vi "dataFGV.vi"(7 "Enum":T1=enum."write data out", 8 "error in (no error)":errorcluster, 10 "DataOut":T3, 11 "DataIn":T2) -> (0 "error out":errorcluster, 2 "DataOut":T3, 3 "DataIn":T2)   [LabVIEW 2017]
uses:
  TypeDefs/dataOut.ctl
  TypeDefs/dataIn.ctl
  TypeDefs/dataFGVState.ctl
  TypeDefs/allData.ctl
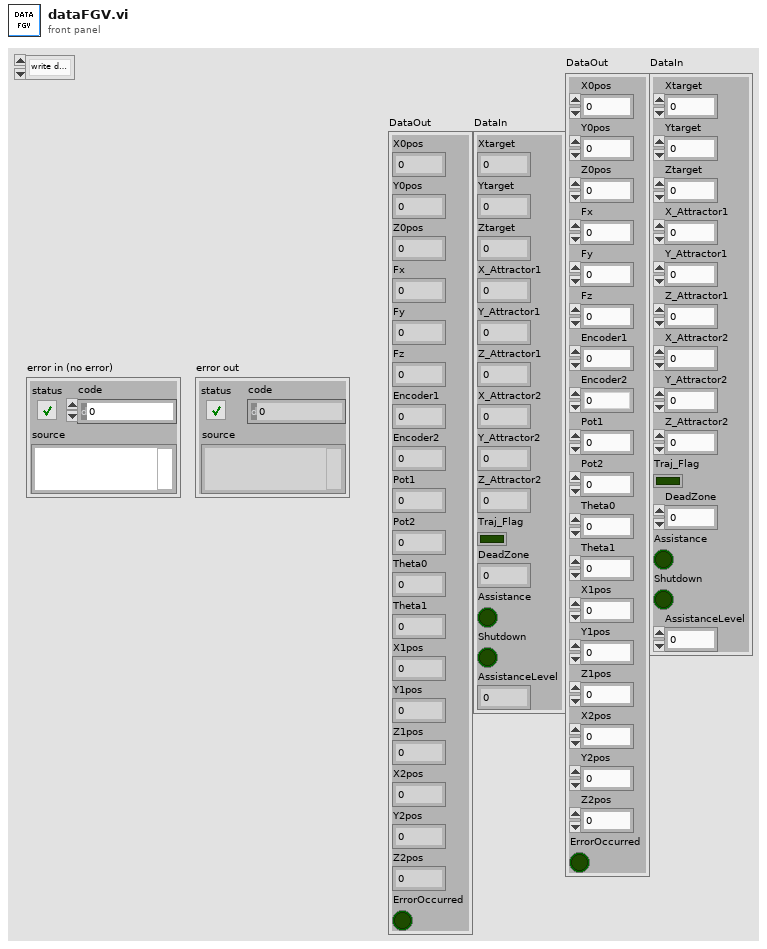
[diagram p1: front panel]
types:
  T1 = typedef "dataFGVState.ctl" = enum16{"init", "write data out", "read data out", "write data in", "read data in"}
  T2 = typedef "dataIn.ctl" = cluster{"Xtarget":dbl, "Ytarget":dbl, "Ztarget":dbl, "X_Attractor1":dbl, "Y_Attractor1":dbl, "Z_Attractor1":dbl, "X_Attractor2":dbl, "Y_Attractor2":dbl, "Z_Attractor2":dbl, "Traj_Flag":bool, "DeadZone":dbl, "Assistance":bool, "Shutdown":bool, "AssistanceLevel":dbl}
  T3 = typedef "dataOut.ctl" = cluster{"X0pos":dbl, "Y0pos":dbl, "Z0pos":dbl, "Fx":dbl, "Fy":dbl, "Fz":dbl, "Encoder1":i32, "Encoder2":i32, "Pot1":dbl, "Pot2":dbl, "Theta0":dbl, "Theta1":dbl, "X1pos":dbl, "Y1pos":dbl, "Z1pos":dbl, "X2pos":dbl, "Y2pos":dbl, "Z2pos":dbl, "ErrorOccurred":bool}
  T4 = typedef "allData.ctl" = cluster{"DataOut":T3, "DataIn":T2}
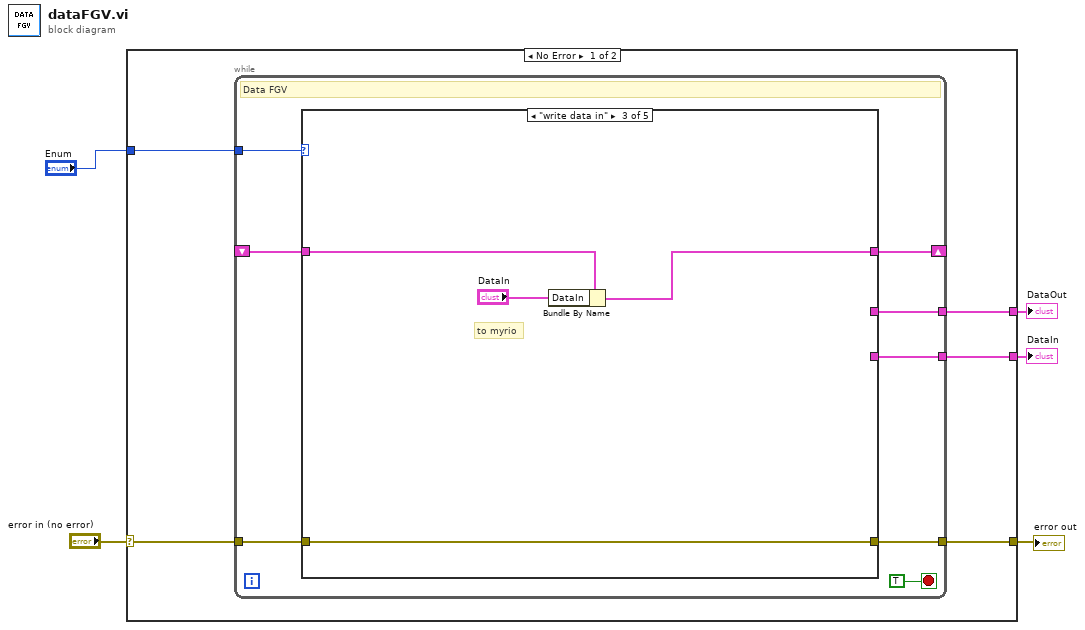
[diagram p0: block diagram]
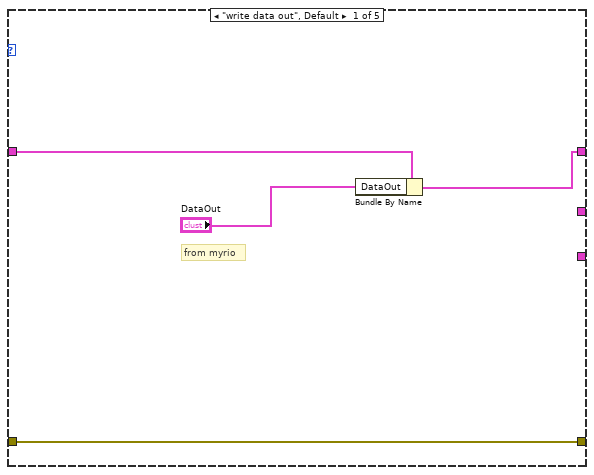
[diagram p2: hidden frame]
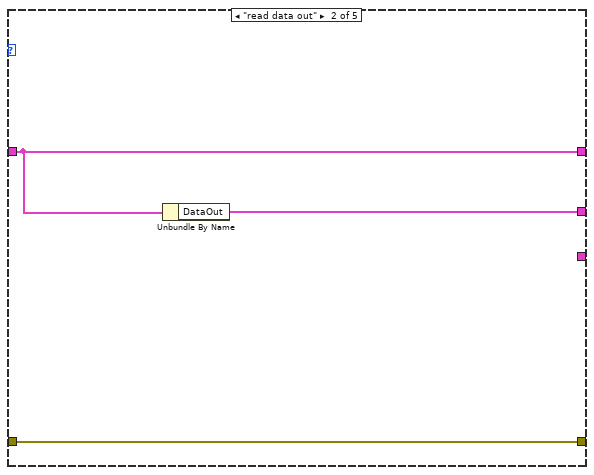
[diagram p3: hidden frame]
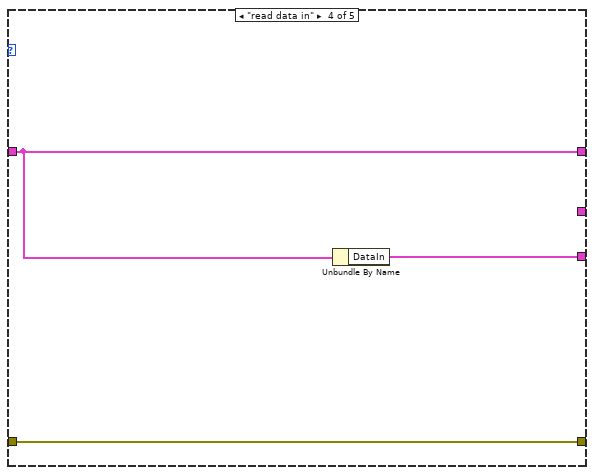
[diagram p4: hidden frame]
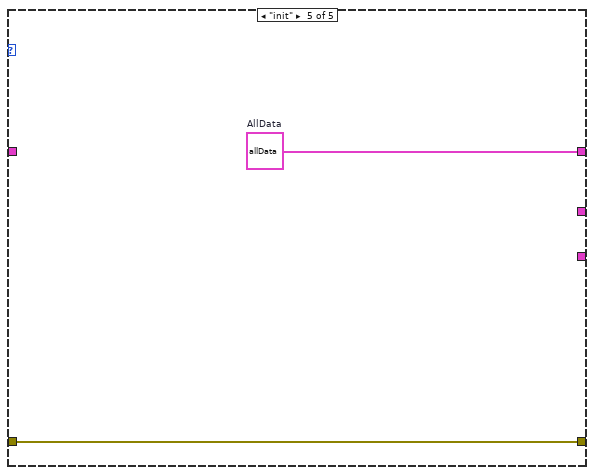
[diagram p5: hidden frame]
diagram:
  n1 = case shown="No Error" "error in (no error)" {
    selector: "error in (no error)" -> [w6 w35]
    tunnel: [w7 w35] -> w4
    tunnel: "Enum" -> [w10 _]
    tunnel: [w9 _] -> w2
    tunnel: [w8 _] -> w1
    frame No Error {
      n2 = while {
        tunnel: w10 -> [w17]
        shift-right: [w16] -> _
        shift-left: _ -> [w15]
        tunnel: [w14] -> w9
        tunnel: [w13] -> w8
        tunnel: [w12] -> w7
        tunnel: w6 -> [w11]
        stop <- TRUE stop-if-true
        # "Data FGV"
        n3 = case shown="\"write data in\"" w17 {
          tunnel: [w21 w25 w28 w31 w34] -> w16
          tunnel: w15 -> [w22 w25 w29 w31 _]
          tunnel: [_ w24 _ _ _] -> w14
          tunnel: [_ _ _ w32 _] -> w13
          tunnel: [w19 w23 w26 w30 w33] -> w12
          tunnel: w11 -> [w19 w23 w26 w30 w33]
          frame "write data out", Default {
            # "from myrio"
            n4 = Bundle By Name(cluster=w22, "DataOut"="DataOut") -> (w21:T4)
          }
          frame "read data out" {
            n5 = Unbundle By Name(w25) -> ("DataOut"=w24:T3)
          }
          frame "write data in" {
            # "to myrio"
            n6 = Bundle By Name(cluster=w29, "DataIn"="DataIn") -> (w28:T4)
          }
          frame "read data in" {
            n7 = Unbundle By Name(w31) -> ("DataIn"=w32:T2)
          }
          frame "init" {
            w34 = T4 {"DataOut"={"X0pos"=0.0, "Y0pos"=0.0, "Z0pos"=0.0, "Fx"=0.0, "Fy"=0.0, "Fz"=0.0, "Encoder1"=0, "Encoder2"=0, "Pot1"=0.0, "Pot2"=0.0, "Theta0"=0.0, "Theta1"=0.0, "X1pos"=0.0, "Y1pos"=0.0, "Z1pos"=0.0, "X2pos"=0.0, "Y2pos"=0.0, "Z2pos"=0.0, "ErrorOccurred"=FALSE}, "DataIn"={"Xtarget"=0.0, "Ytarget"=0.0, "Ztarget"=0.0, "X_Attractor1"=0.0, "Y_Attractor1"=0.0, "Z_Attractor1"=0.0, "X_Attractor2"=0.0, "Y_Attractor2"=0.0, "Z_Attractor2"=0.0, "Traj_Flag"=FALSE, "DeadZone"=0.0, "Assistance"=FALSE, "Shutdown"=FALSE, "AssistanceLevel"=0.0}}  # AllData
          }
        }
      }
    }
    frame Error {
    }
  }
  "error out" <- w4
  "DataOut" <- w2
  "DataIn" <- w1
